vi "Get current activity.vi"(8 "error in (no error)":errorcluster, 11 "Tomo in":refnum<class "Tomo.lvclass">) -> (0 "error out":errorcluster, 2 "Current activity":T1, 3 "Tomo out":refnum<class "Tomo.lvclass">)   [LabVIEW 2012, in "Tomo.lvclass"]
uses:
  Tomo.lvclass
  Current activity.ctl
  Tomo.lvclass/Tomo.ctl
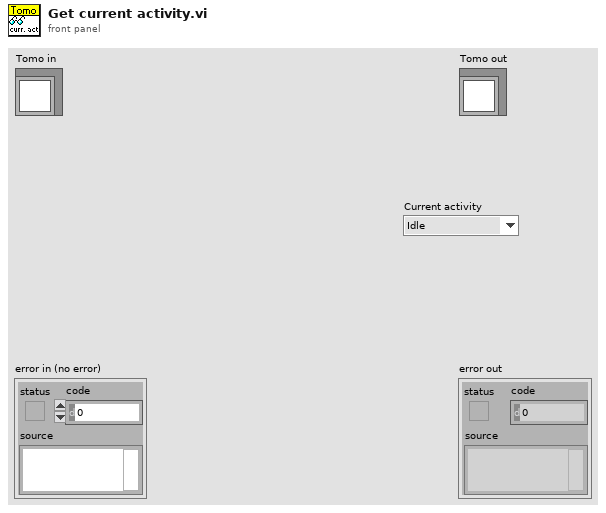
[diagram p1: front panel]
types:
  T1 = typedef "Tomo.lvclass/Current activity.ctl" = enum16{"Idle", "Inter-stack motion", "Pre-tomo calculation", "Stack acquisition", "Stack preparation", "Pre-tomo stack acq", "Pre-tomo inter-stack"}
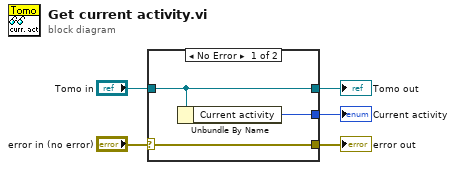
[diagram p0: block diagram]
diagram:
  n1 = case shown="No Error" "error in (no error)" {
    selector: "error in (no error)" -> [w8 w10]
    tunnel: [w8 w10] -> w4
    tunnel: [w7 w9] -> w2
    tunnel: "Tomo in" -> [w7 w9]
    tunnel: [w6 _] -> w1
    frame No Error {
      n2 = Unbundle By Name(w7) -> ("Current activity"=w6:T1)
    }
    frame Error {
    }
  }
  "error out" <- w4
  "Tomo out" <- w2
  "Current activity" <- w1
